vi "配置文件读取写入.vi"(7 "配置模式":enum16{"读取", "写入"}(ring), 8 "error in (no error)":errorcluster caption="错误输入（无错误）", 10 "配置文件名":string, 11 "配置信息":T8) -> (0 "error out":errorcluster caption="错误输出", 3 "配置信息读取":T8)   [LabVIEW 2016, in "定时设置.xctl"]
uses:
  <vilib>/Utility/xml.llb/Read From XML File(string).vi
  <vilib>/Utility/xml.llb/Write to XML File(string).vi
panel:
  # "分钟"
  # "次"
  # "分钟"
  # "次"
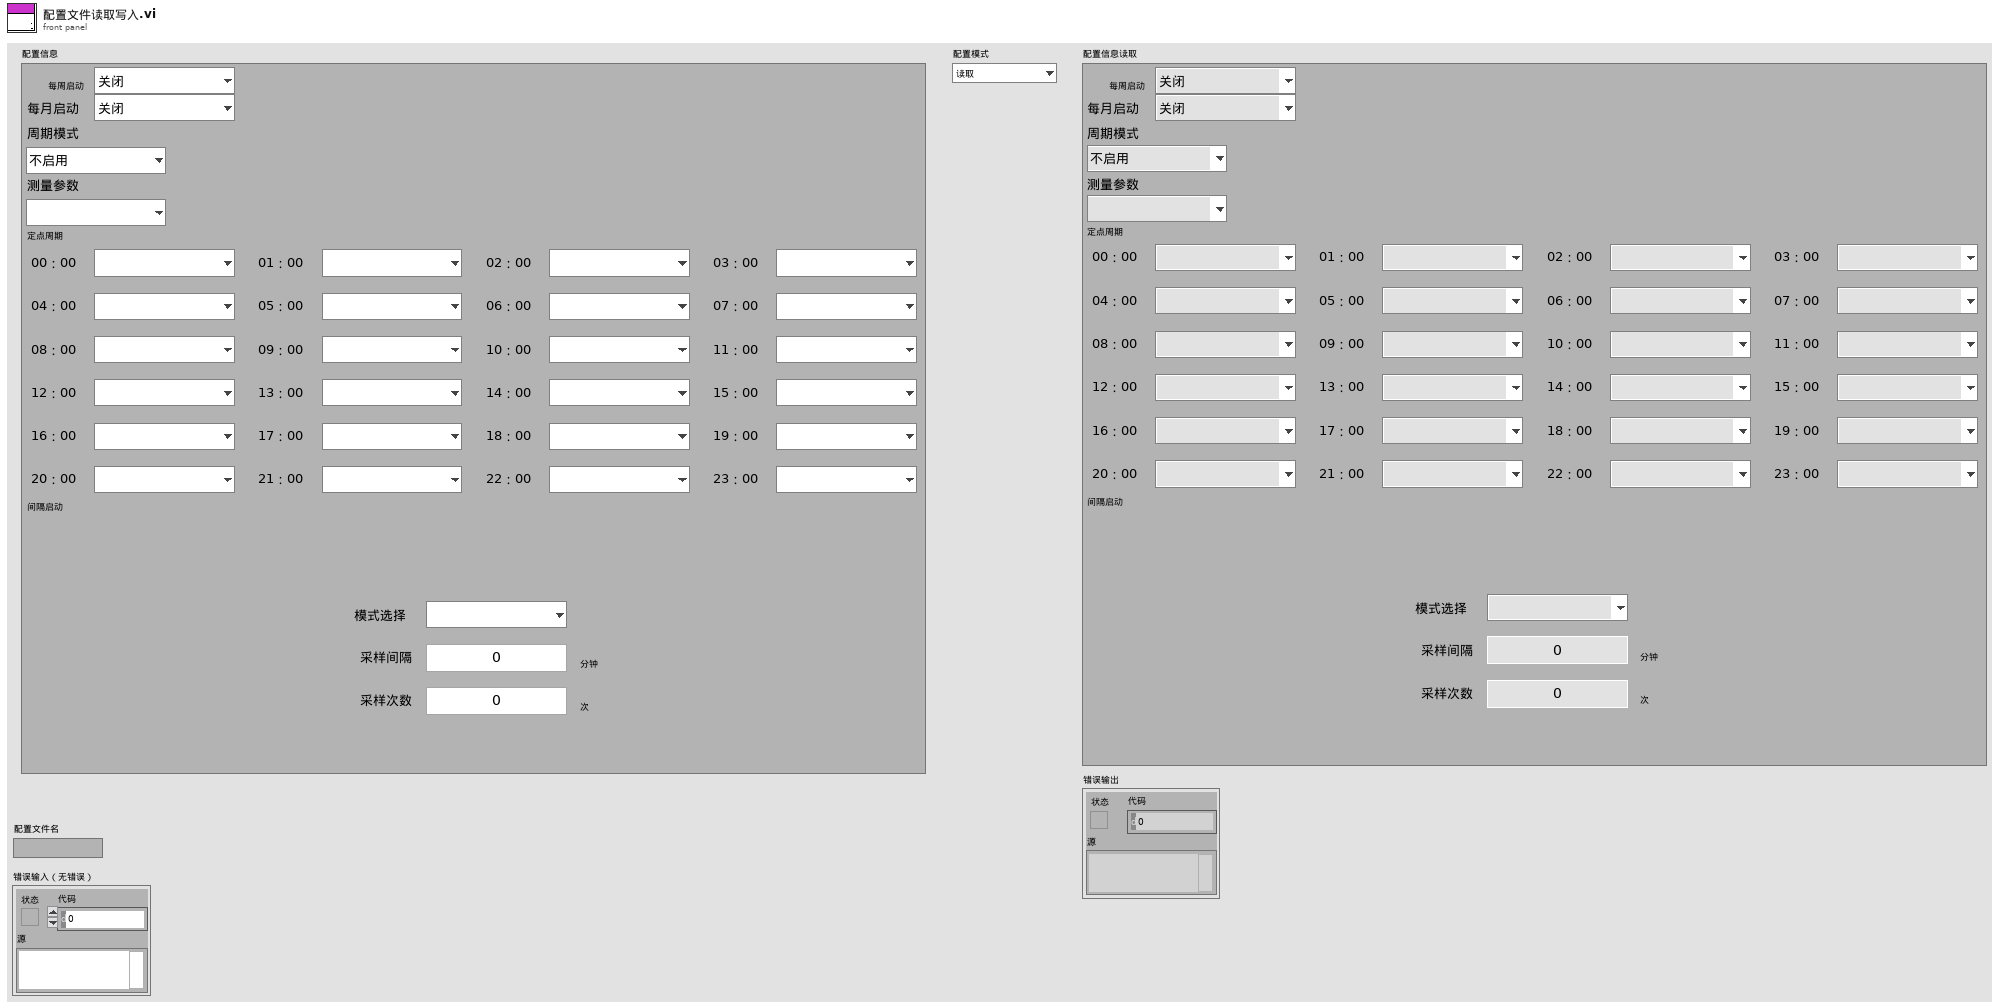
[diagram p1: front panel]
types:
  T1 = typedef "定时设置.xctl/每周启动.ctl" = enum16{"关闭", "周日", "周一", "周二", "周三", "周四", "周五", "周六"}
  T2 = typedef "定时设置.xctl/每月启动.ctl" = enum16{"关闭", "1号", "2号", "3号", "4号", "5号", "6号", "7号", "8号", "9号", "10号", "11号", "12号", "13号", "14号", "15号", "16号", "17号", "18号", "19号", "20号", "21号", "22号", "23号", "24号", "25号", "26号", "27号", "28号", "29号", "30号", "31号"}
  T3 = typedef "定时设置.xctl/周期模式设置.ctl" = enum16{"不启用", "定点模式", "间隔模式"}
  T4 = typedef "定时设置.xctl/测量参数.ctl" = u16
  T5 = typedef "定时设置.xctl/定点周期设置.ctl" = cluster{"启动命令":T6, "启动命令 2":T6, "启动命令 3":T6, "启动命令 4":T6, "启动命令 5":T6, "启动命令 6":T6, "启动命令 7":T6, "启动命令 8":T6, "启动命令 9":T6, "启动命令 10":T6, "启动命令 11":T6, "启动命令 12":T6, "启动命令 13":T6, "启动命令 14":T6, "启动命令 15":T6, "启动命令 16":T6, "启动命令 17":T6, "启动命令 18":T6, "启动命令 19":T6, "启动命令 20":T6, "启动命令 21":T6, "启动命令 22":T6, "启动命令 23":T6, "启动命令 24":T6}
  T6 = typedef "定时设置.xctl/启动命令选择.ctl" = enum16{"", "水样测试", "标样核查", "零点核查", "跨度核查", "空白测试", "平行样测试", "加标回收", "空白校准", "标样校准", "初始化(清洗)"}
  T7 = typedef "定时设置.xctl/间隔启动设置.ctl" = cluster{"启动命令":T6, "启动间隔":dbl, "启动次数":i32}
  T8 = cluster{"每周启动":T1, "每月启动":T2, "周期模式":T3, "测量参数":T4, "定点周期":T5, "间隔启动":T7}
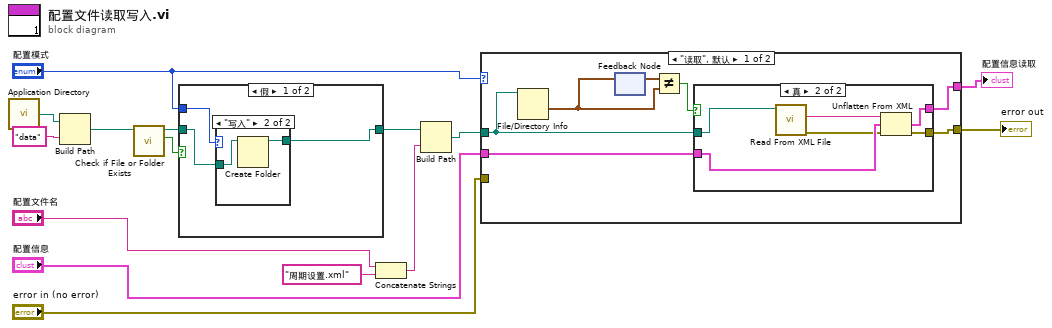
[diagram p0: block diagram]
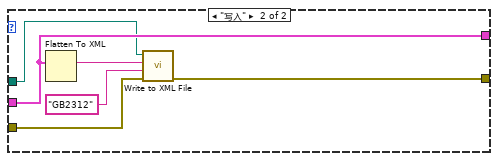
[diagram p3: hidden frame]
diagram:
  n1 = call <vilib>:"Application Directory.vi"() -> ("Application Directory"=w15:path)
  n2 = Build Path(base path=w15, name or relative path="data" ("名称或相对路径")) -> (appended path=w13:path)
  n3 = call <vilib>:"Check if File or Folder Exists.vi"("path"=w13) -> ("file or folder exists?"=w11:bool, "dup path"=w12:path)  [unwired: 8 in, 1 out]
  n4 = case shown="假" w11 {
    tunnel: w12 -> [w18 w22]
    tunnel: [w17 w22] -> w10
    tunnel: "配置模式" -> [w16 _]
    frame False {
      n5 = case shown="\"写入\"" w16 {
        tunnel: w18 -> [w19 w21]
        tunnel: [w19 w20] -> w17
        frame "读取", Default {
        }
        frame "写入" {
          n6 = Create Folder(path (use dialog)=w21) -> (created path=w20:path)  [unwired: 2 in, 2 out]
        }
      }
    }
    frame True {
    }
  }
  n7 = Concatenate Strings("配置文件名", "周期设置.xml" ("字符串")) -> (w8:string)
  n8 = Build Path(base path=w10, name or relative path=w8) -> (appended path=w4:path)
  n9 = case shown="\"读取\", 默认" "配置模式" {
    tunnel: "配置信息" -> [w29 w42]
    tunnel: [w27 w37] -> w2
    tunnel: [w28 w42] -> w5
    tunnel: w4 -> [w26 w41]
    tunnel: "error in (no error)" -> [_ w39]
    frame "读取", Default {
      n10 = File/Directory Info(path=w26) -> (last mod=w24:timestamp)  [unwired: 1 in, 6 out]
      n11 = feedback-in #1(w24) -> ()
      n12 = feedback #1() -> (w25:timestamp)  [unwired: 1 in]
      n13 = Not Equal?(x=w25, y=w24) -> (x != y?=w23:bool)
      n14 = case shown="真" w23 {
        tunnel: w29 -> [w30 w35]
        tunnel: [w30 w34] -> w28
        tunnel: [_ w33] -> w27
        tunnel: w26 -> [_ w31]
        frame False {
        }
        frame True {
          n15 = call-poly <vilib>:"Read From XML File.vi"("XML File Path"=w31) -> ("error out"=w32:errorcluster, "XML Elements"=w36:string)  [unwired: 8 in, 1 out]
          n16 = Unflatten From XML(xml string=w36, type=w35, error in (no error)=w32) -> (value=w34:T8, error out=w33:errorcluster)
        }
      }
    }
    frame "写入" {
      n17 = Flatten To XML(anything=w42) -> (xml string=w40:string)
      n18 = call-poly <vilib>:"Write to XML File.vi"("error in (no error)"=w39, "XML Encoding"="GB2312", "XML Input"=w40, "XML File Path"=w41) -> ("error out"=w37:errorcluster)  [unwired: 5 in, 2 out]
    }
  }
  "配置信息读取" <- w5
  "error out" <- w2
